vi "_ConvertLensTable.vi"(4 "UseESI1":bool, 5 "IsNegative":bool, 6 "MethodLevelParameters":string[][](array[string]), 7 "Expt":string[](array[string]), 8 "ExptParamAndMR":T3) -> (2 "LensTable":T1[](array[typedef]))   [LabVIEW 2015]
uses:
  Type/_Mass Range Parameters.ctl
  Type/_Lens Property.ctl
  Configuration/_Global Configuration.vi
panel:
  # "Num             Type            Polarity        StartTime      StopTime        Cycles       PauseTime    DelayTime          MR#         DwellTime   Comment"
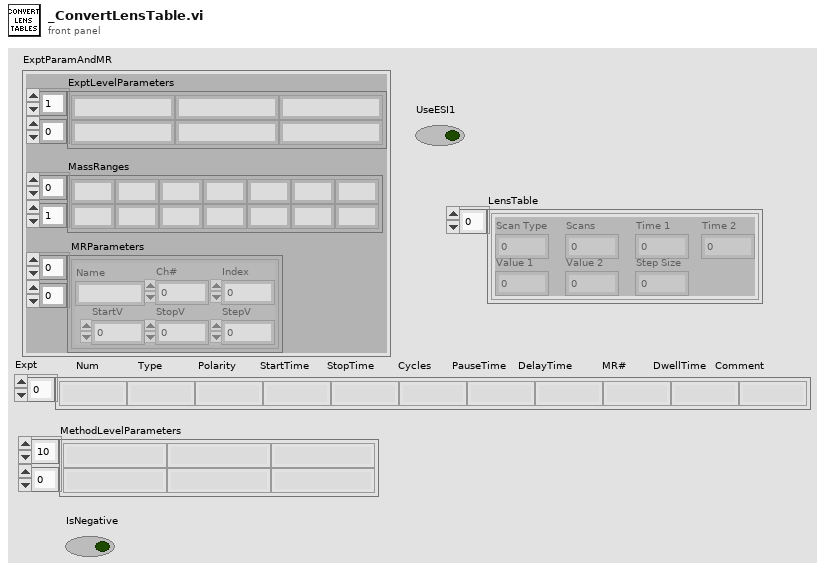
[diagram p1: front panel]
types:
  T1 = typedef "_Lens Property.ctl" = cluster{"Scan Type":u8, "Scans":i32, "Time 1":dbl, "Time 2":dbl, "Value 1":dbl, "Value 2":dbl, "Step Size":dbl}
  T2 = typedef "_Mass Range Parameters.ctl" = cluster{"Name":string, "Ch#":u8, "StartV":dbl, "StopV":dbl, "StepV":dbl, "Index":u8}
  T3 = cluster{"ExptLevelParameters":string[][], "MassRanges":string[][], " MRParameters":T2[][]}
  T4 = typedef "_RT Instrument 2.ctl" = cluster{"Table":T5[], "Instrument":string[]}
  T5 = typedef "_RT Configuration 2.ctl" = cluster{"Name":string, "Ch#":u8, "Min":dbl, "Max":dbl, "Def+":dbl, "Def-":dbl, "Offset":dbl, "Slope":dbl, "Type":u8, "Description":string, "SettleT":dbl}
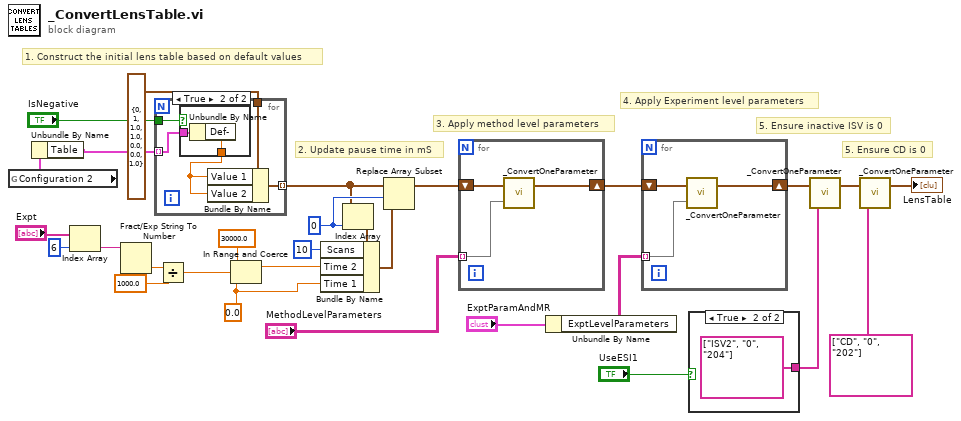
[diagram p0: block diagram]
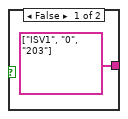
[diagram p2: hidden frame]
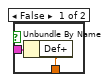
[diagram p3: hidden frame]
diagram:
  w15 = 0.0 ("lower limit")
  w24 = 0 ("index")
  # "5. Ensure CD is 0"
  # "5. Ensure inactive ISV is 0"
  # "4. Apply Experiment level parameters"
  # "3. Apply method level parameters"
  # "2. Update pause time in mS"
  # "1. Construct the initial lens table based on default values"
  n1 = global read "_Global Configuration.vi" "Configuration 2"() -> (w29:T4)
  n2 = Unbundle By Name(w29) -> ("Table"=w26:T5[])
  n3 = Index Array(array="Expt", index=6) -> (element=w18:string)
  n4 = Fract/Exp String To Number(string=w18) -> (number=w14:dbl)  [unwired: 3 in, 1 out]
  n5 = for {
    tunnel: w26 -> [w33] mode=indexing
    tunnel: T1 {"Scan Type"=0, "Scans"=1, "Time 1"=1.0, "Time 2"=1.0, "Value 1"=0.0, "Value 2"=0.0, "Step Size"=1.0} ("Lenses") -> [w34]
    tunnel: [w32] -> w22 mode=indexing
    tunnel: "IsNegative" -> [w31]
    n6 = case shown="True" w31 {
      tunnel: w33 -> [w36 w38]
      tunnel: [w35 w37] -> w30
      frame False {
        n7 = Unbundle By Name(w36) -> ("Def+"=w35:dbl)
      }
      frame True {
        n8 = Unbundle By Name(w38) -> ("Def-"=w37:dbl)
      }
    }
    n9 = Bundle By Name(cluster=w34, "Value 1"=w30, "Value 2"=w30) -> (w32:T1)
  }
  n10 = Divide(x=w14, y=1000.0) -> (x/y=w12:dbl)
  n11 = In Range and Coerce(upper limit=30000.0, x=w12, lower limit=w15) -> (coerced(x)=w16:dbl)  [unwired: 1 out]
  n12 = Index Array(array=w22, index=w24) -> (element=w23:T1)
  n13 = Bundle By Name(cluster=w23, "Scans"=10, "Time 2"=w16, "Time 1"=w15) -> (w25:T1)
  n14 = Replace Array Subset(array=w22, new element=w25, index=w24) -> (w11:T1[])
  n15 = for {
    shift-right: [w40] -> w8
    shift-left: w11 -> [w39]
    tunnel: "MethodLevelParameters" -> [w41] mode=indexing
    n16 = call "_ConvertOneParameter.vi"("Parameter"=w41, "LensTableIn"=w39) -> ("LensTableOut"=w40:T1[])  [unwired: 1 out]
  }
  n17 = Unbundle By Name("ExptParamAndMR") -> ("ExptLevelParameters"=w7:string[][])
  n18 = for {
    shift-right: [w43] -> w6
    shift-left: w8 -> [w42]
    tunnel: w7 -> [w44] mode=indexing
    n19 = call "_ConvertOneParameter.vi"("Parameter"=w44, "LensTableIn"=w42) -> ("LensTableOut"=w43:T1[])  [unwired: 1 out]
  }
  n20 = case shown="True" "UseESI1" {
    tunnel: [string[] ["ISV1", "0", "203"] ("Parameter") string[] ["ISV2", "0", "204"] ("Parameter")] -> w5
    frame False {
    }
    frame True {
    }
  }
  n21 = call "_ConvertOneParameter.vi"("Parameter"=w5, "LensTableIn"=w6) -> ("LensTableOut"=w3:T1[])  [unwired: 1 out]
  n22 = call "_ConvertOneParameter.vi"("Parameter"=string[] ["CD", "0", "202"], "LensTableIn"=w3) -> ("LensTableOut"=→"LensTable":T1[])  [unwired: 1 out]
